vi "Modbus LDO Sensors.vi"(8 "error in":errorcluster, 11 "PLC Data":T1) -> (0 "error out":errorcluster, 3 "PLC Data Output":T1)   [LabVIEW 2020, in "Modbus.lvlib"]
uses:
  Modbus.lvlib
  Modbus PLC Data All.ctl
  Modbus FVIR Control.ctl
  Modbus LDO Control.ctl
  WritingDataFile/Data to Save.ctl
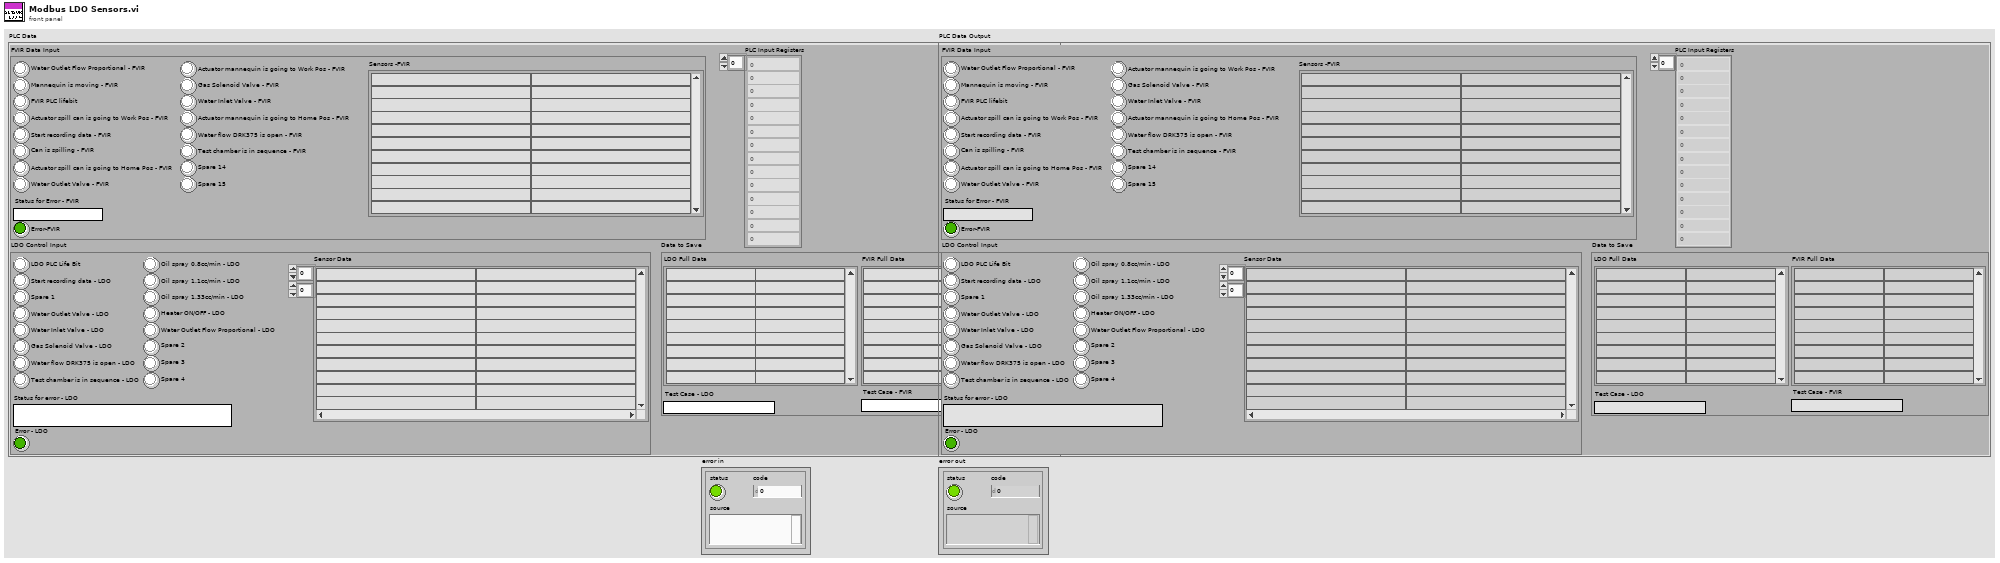
[diagram p1: front panel]
types:
  T1 = typedef "Modbus PLC Data All.ctl" = cluster{"FVIR Data Input":T2, "LDO Control Input":T3, "PLC Input Registers":u16[], "Data to Save":T4}
  T2 = typedef "Modbus FVIR Control.ctl" = cluster{"Spare 15":bool, "Spare 14":bool, "Actuator mannequin is going to Work Pos - FVIR":bool, "Actuator mannequin is going to Home Pos - FVIR":bool, "Test chamber is in sequence - FVIR ":bool, "Water flow DRK375 is open - FVIR":bool, "Gas Solenoid Valve - FVIR":bool, "Water Inlet Valve - FVIR":bool, "Water Outlet Flow Proportional - FVIR":bool, "Start recording data - FVIR":bool, "Actuator spill can is going to Work Pos - FVIR":bool, "Actuator spill can is going to Home Pos - FVIR":bool, "Water Outlet Valve - FVIR":bool, "Can is spilling - FVIR":bool, "Mannequin is moving - FVIR":bool, "FVIR PLC lifebit":bool, "Status for Error - FVIR":string, "Error-FVIR":bool, "Sensors -FVIR":string[][]}
  T3 = typedef "Modbus LDO Control.ctl" = cluster{"LDO PLC Life Bit":bool, "Start recording data - LDO":bool, "Spare 1":bool, "Water Outlet Valve - LDO":bool, "Water Inlet Valve - LDO":bool, "Gas Solenoid Valve - LDO":bool, "Water flow DRK375 is open - LDO":bool, "Test chamber is in sequence - LDO":bool, "Oil spray 0.8cc/min - LDO":bool, "Oil spray 1.1cc/min - LDO":bool, "Oil spray 1.33cc/min - LDO":bool, "Heater ON/OFF - LDO":bool, "Water Outlet Flow Proportional - LDO":bool, "Spare 2":bool, "Spare 3":bool, "Spare 4":bool, "Status for error - LDO":string, "Error - LDO":bool, "Sensor Data":string[][]}
  T4 = typedef "Data to Save.ctl" = cluster{"LDO Full Data":string[][], "FVIR Full Data":string[][], "Test Case - FVIR":string, "Test Case - LDO":string}
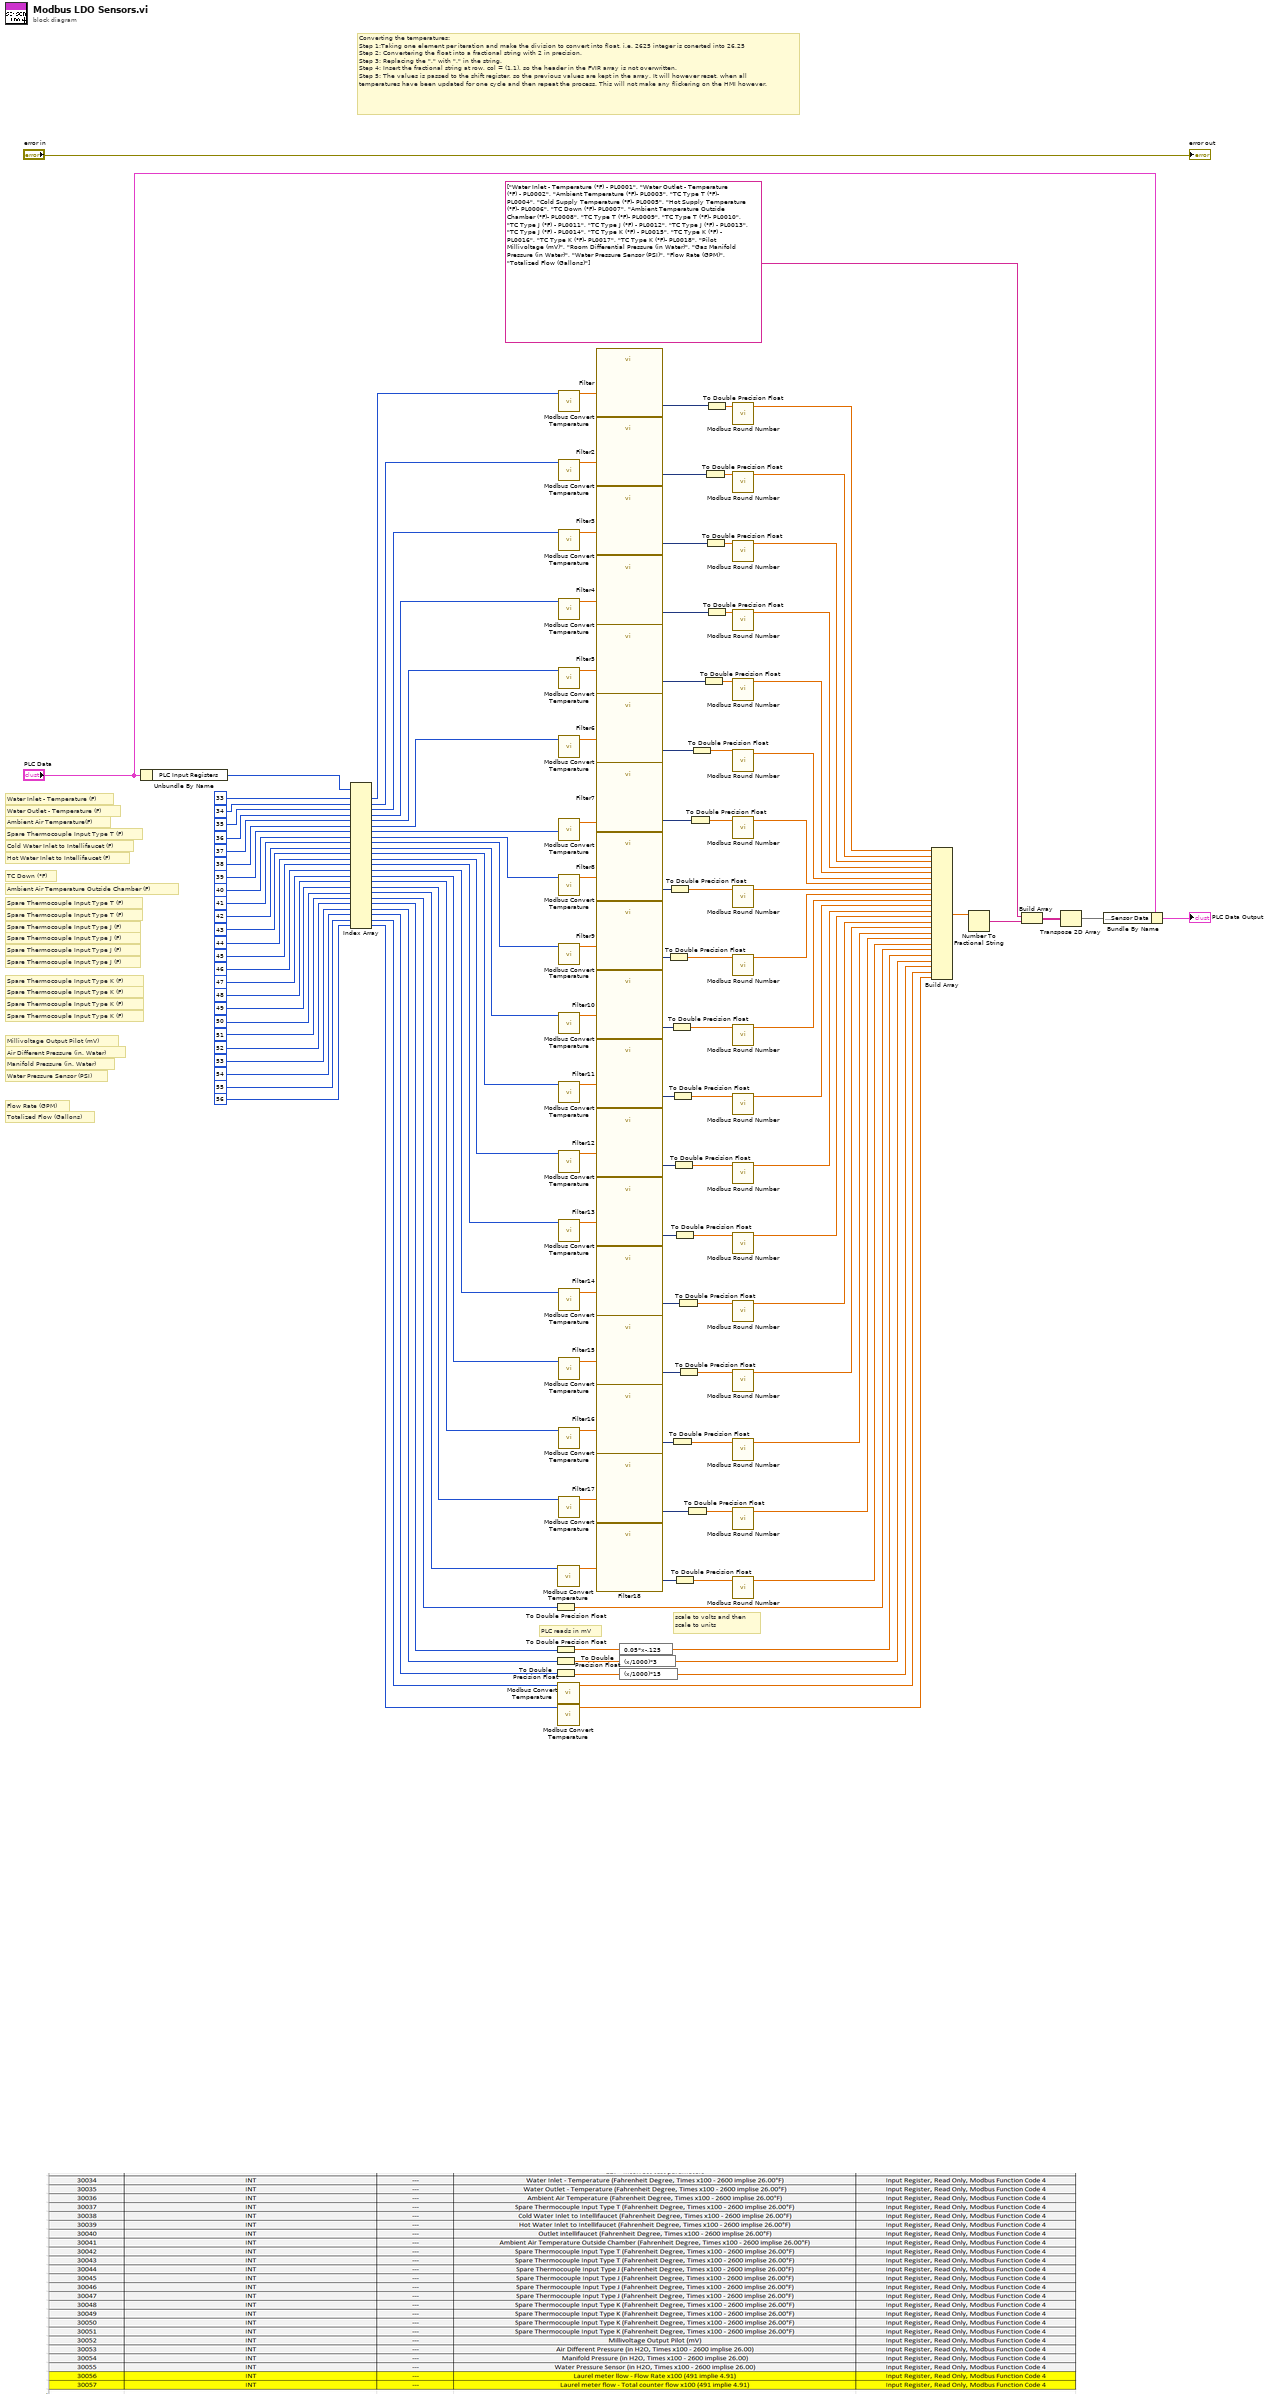
[diagram p0: block diagram]
diagram:
  # "scale to volts and then \nscale to units"
  # "PLC reads in mV"
  # "Totalized Flow (Gallons)"
  # "Flow Rate (GPM)"
  # "Water Pressure Sensor (PSI)"
  # "Manifold Pressure (in. Water)"
  # "Air Different Pressure (in. Water)"
  # "Millivoltage Output Pilot (mV)"
  # "Spare Thermocouple Input Type K (F)"
  # "Spare Thermocouple Input Type K (F)"
  # "Spare Thermocouple Input Type K (F)"
  # "Spare Thermocouple Input Type K (F)"
  # "Spare Thermocouple Input Type J (F)"
  # "Spare Thermocouple Input Type J (F)"
  # "Spare Thermocouple Input Type J (F)"
  # "Spare Thermocouple Input Type J (F)"
  # "Spare Thermocouple Input Type T (F)"
  # "Spare Thermocouple Input Type T (F)"
  # "Ambient Air Temperature Outside Chamber (F)"
  # "TC Down (°F)"
  # "Hot Water Inlet to Intellifaucet (F)"
  # "Cold Water Inlet to Intellifaucet (F)"
  # "Spare Thermocouple Input Type T (F)"
  # "Ambient Air Temperature(F)"
  # "Water Outlet - Temperature (F)"
  # "Water Inlet - Temperature (F)"
  # "Converting the temperatures: \nStep 1:Taking one element per iteration and make the division to convert into float, i.e. 2625 integer is conerted into 26,25\nStep 2: Convertering the float into a fractional string with 2 in precision. \nStep 3: Replacing the \",\" with \".\" in the string.\nStep 4: Insert the fractional string at row, col = (1,1), so the header in the FVIR array is not overwritten. \nStep 5: The values is passed to the shift register, so the previous values are kept in the array. It will however reset, when all temperatures have been updated for one cycle and then repeat the process. This will not make any flickering on the HMI however."
  n1 = Unbundle By Name("PLC Data") -> ("PLC Input Registers"=w82:u16[])
  n2 = Index Array(array=w82, index #1=33 ("index"), index #2=34 ("index"), index #3=35 ("index"), index #4=36 ("index"), index #5=37 ("index"), index #6=38 ("index"), index #7=39 ("index"), index #8=40 ("index"), index #9=41 ("index"), index #10=42 ("index"), index #11=43 ("index"), index #12=44 ("index"), index #13=45 ("index"), index #14=46 ("index"), index #15=47 ("index"), index #16=48 ("index"), index #17=49 ("index"), index #18=50 ("index"), index #19=51 ("index"), index #20=52 ("index"), index #21=53 ("index"), index #22=54 ("index"), index #23=55 ("index"), index #24=56 ("index")) -> (element #1=w114:u16, element #2=w113:u16, element #3=w112:u16, element #4=w111:u16, element #5=w110:u16, element #6=w109:u16, element #7=w108:u16, element #8=w107:u16, element #9=w106:u16, element #10=w105:u16, element #11=w104:u16, element #12=w103:u16, element #13=w102:u16, element #14=w101:u16, element #15=w100:u16, element #16=w99:u16, element #17=w98:u16, element #18=w97:u16, element #19=w74:u16, element #20=w95:u16, element #21=w81:u16, element #22=w94:u16, element #23=w93:u16, element #24=w92:u16)
  n3 = To Double Precision Float(number=w74) -> (double precision float=w73:dbl)
  n4 = To Double Precision Float(number=w95) -> (double precision float=w79:dbl)
  n5 = To Double Precision Float(number=w81) -> (double precision float=w80:dbl)
  n6 = To Double Precision Float(number=w94) -> (double precision float=w76:dbl)
  n7 = call "Modbus Convert Temperature.vi"("PLC Value"=w97) -> ("Converted Value"=w37:dbl)  [unwired: 9 in, 1 out]
  n8 = call "Modbus Convert Temperature.vi"("PLC Value"=w93) -> ("Converted Value"=w91:dbl)  [unwired: 9 in, 1 out]
  n9 = call "Modbus Convert Temperature.vi"("PLC Value"=w92) -> ("Converted Value"=w90:dbl)  [unwired: 9 in, 1 out]
  n10 = call "Modbus Convert Temperature.vi"("PLC Value"=w114) -> ("Converted Value"=w72:dbl)  [unwired: 9 in, 1 out]
  n11 = call "Modbus Convert Temperature.vi"("PLC Value"=w113) -> ("Converted Value"=w69:dbl)  [unwired: 9 in, 1 out]
  n12 = call "Modbus Convert Temperature.vi"("PLC Value"=w112) -> ("Converted Value"=w67:dbl)  [unwired: 9 in, 1 out]
  n13 = call "Modbus Convert Temperature.vi"("PLC Value"=w111) -> ("Converted Value"=w65:dbl)  [unwired: 9 in, 1 out]
  n14 = call "Modbus Convert Temperature.vi"("PLC Value"=w110) -> ("Converted Value"=w63:dbl)  [unwired: 9 in, 1 out]
  n15 = call "Modbus Convert Temperature.vi"("PLC Value"=w109) -> ("Converted Value"=w61:dbl)  [unwired: 9 in, 1 out]
  n16 = call "Modbus Convert Temperature.vi"("PLC Value"=w108) -> ("Converted Value"=w59:dbl)  [unwired: 9 in, 1 out]
  n17 = call "Modbus Convert Temperature.vi"("PLC Value"=w107) -> ("Converted Value"=w57:dbl)  [unwired: 9 in, 1 out]
  n18 = call "Modbus Convert Temperature.vi"("PLC Value"=w106) -> ("Converted Value"=w55:dbl)  [unwired: 9 in, 1 out]
  n19 = call "Modbus Convert Temperature.vi"("PLC Value"=w105) -> ("Converted Value"=w53:dbl)  [unwired: 9 in, 1 out]
  n20 = call "Modbus Convert Temperature.vi"("PLC Value"=w104) -> ("Converted Value"=w51:dbl)  [unwired: 9 in, 1 out]
  n21 = call "Modbus Convert Temperature.vi"("PLC Value"=w103) -> ("Converted Value"=w49:dbl)  [unwired: 9 in, 1 out]
  n22 = call "Modbus Convert Temperature.vi"("PLC Value"=w102) -> ("Converted Value"=w47:dbl)  [unwired: 9 in, 1 out]
  n23 = call "Modbus Convert Temperature.vi"("PLC Value"=w101) -> ("Converted Value"=w45:dbl)  [unwired: 9 in, 1 out]
  n24 = call "Modbus Convert Temperature.vi"("PLC Value"=w100) -> ("Converted Value"=w43:dbl)  [unwired: 9 in, 1 out]
  n25 = call "Modbus Convert Temperature.vi"("PLC Value"=w99) -> ("Converted Value"=w41:dbl)  [unwired: 9 in, 1 out]
  n26 = call "Modbus Convert Temperature.vi"("PLC Value"=w98) -> ("Converted Value"=w39:dbl)  [unwired: 9 in, 1 out]
  n27 = call "Filter"("Signal"=w72) -> ("Filtered Signal"=w71:dynamicdata)  [unwired: 9 in, 1 out]
  n28 = call "Filter2"("Signal"=w69) -> ("Filtered Signal"=w70:dynamicdata)  [unwired: 9 in, 1 out]
  n29 = call "Filter3"("Signal"=w67) -> ("Filtered Signal"=w68:dynamicdata)  [unwired: 9 in, 1 out]
  n30 = call "Filter4"("Signal"=w65) -> ("Filtered Signal"=w66:dynamicdata)  [unwired: 9 in, 1 out]
  n31 = call "Filter5"("Signal"=w63) -> ("Filtered Signal"=w64:dynamicdata)  [unwired: 9 in, 1 out]
  n32 = call "Filter6"("Signal"=w61) -> ("Filtered Signal"=w62:dynamicdata)  [unwired: 9 in, 1 out]
  n33 = call "Filter7"("Signal"=w59) -> ("Filtered Signal"=w60:dynamicdata)  [unwired: 9 in, 1 out]
  n34 = call "Filter8"("Signal"=w57) -> ("Filtered Signal"=w58:dynamicdata)  [unwired: 9 in, 1 out]
  n35 = call "Filter9"("Signal"=w55) -> ("Filtered Signal"=w56:dynamicdata)  [unwired: 9 in, 1 out]
  n36 = call "Filter10"("Signal"=w53) -> ("Filtered Signal"=w54:dynamicdata)  [unwired: 9 in, 1 out]
  n37 = call "Filter11"("Signal"=w51) -> ("Filtered Signal"=w52:dynamicdata)  [unwired: 9 in, 1 out]
  n38 = call "Filter12"("Signal"=w49) -> ("Filtered Signal"=w50:dynamicdata)  [unwired: 9 in, 1 out]
  n39 = call "Filter13"("Signal"=w47) -> ("Filtered Signal"=w48:dynamicdata)  [unwired: 9 in, 1 out]
  n40 = call "Filter14"("Signal"=w45) -> ("Filtered Signal"=w46:dynamicdata)  [unwired: 9 in, 1 out]
  n41 = call "Filter15"("Signal"=w43) -> ("Filtered Signal"=w44:dynamicdata)  [unwired: 9 in, 1 out]
  n42 = call "Filter16"("Signal"=w41) -> ("Filtered Signal"=w42:dynamicdata)  [unwired: 9 in, 1 out]
  n43 = call "Filter17"("Signal"=w39) -> ("Filtered Signal"=w40:dynamicdata)  [unwired: 9 in, 1 out]
  n44 = call "Filter18"("Signal"=w37) -> ("Filtered Signal"=w38:dynamicdata)  [unwired: 9 in, 1 out]
  n45 = expression code="0.05*x-.125"(w79) -> (w78:dbl)
  n46 = expression code="(x/1000)*3"(w80) -> (w77:dbl)
  n47 = expression code="(x/1000)*15"(w76) -> (w75:dbl)
  n48 = To Double Precision Float(number=w56) -> (double precision float=w20:dbl)
  n49 = To Double Precision Float(number=w58) -> (double precision float=w22:dbl)
  n50 = To Double Precision Float(number=w54) -> (double precision float=w18:dbl)
  n51 = To Double Precision Float(number=w42) -> (double precision float=w6:dbl)
  n52 = To Double Precision Float(number=w52) -> (double precision float=w16:dbl)
  n53 = To Double Precision Float(number=w50) -> (double precision float=w14:dbl)
  n54 = To Double Precision Float(number=w48) -> (double precision float=w12:dbl)
  n55 = To Double Precision Float(number=w38) -> (double precision float=w2:dbl)
  n56 = To Double Precision Float(number=w46) -> (double precision float=w10:dbl)
  n57 = To Double Precision Float(number=w44) -> (double precision float=w8:dbl)
  n58 = To Double Precision Float(number=w40) -> (double precision float=w4:dbl)
  n59 = To Double Precision Float(number=w60) -> (double precision float=w24:dbl)
  n60 = To Double Precision Float(number=w62) -> (double precision float=w26:dbl)
  n61 = To Double Precision Float(number=w64) -> (double precision float=w28:dbl)
  n62 = To Double Precision Float(number=w70) -> (double precision float=w34:dbl)
  n63 = To Double Precision Float(number=w68) -> (double precision float=w32:dbl)
  n64 = To Double Precision Float(number=w71) -> (double precision float=w36:dbl)
  n65 = To Double Precision Float(number=w66) -> (double precision float=w30:dbl)
  n66 = call "Modbus Round Number.vi"("Number"=w36) -> ("Rounded Number"=w35:dbl)  [unwired: 10 in]
  n67 = call "Modbus Round Number.vi"("Number"=w34) -> ("Rounded Number"=w33:dbl)  [unwired: 10 in]
  n68 = call "Modbus Round Number.vi"("Number"=w32) -> ("Rounded Number"=w31:dbl)  [unwired: 10 in]
  n69 = call "Modbus Round Number.vi"("Number"=w30) -> ("Rounded Number"=w29:dbl)  [unwired: 10 in]
  n70 = call "Modbus Round Number.vi"("Number"=w28) -> ("Rounded Number"=w27:dbl)  [unwired: 10 in]
  n71 = call "Modbus Round Number.vi"("Number"=w26) -> ("Rounded Number"=w25:dbl)  [unwired: 10 in]
  n72 = call "Modbus Round Number.vi"("Number"=w24) -> ("Rounded Number"=w23:dbl)  [unwired: 10 in]
  n73 = call "Modbus Round Number.vi"("Number"=w22) -> ("Rounded Number"=w21:dbl)  [unwired: 10 in]
  n74 = call "Modbus Round Number.vi"("Number"=w20) -> ("Rounded Number"=w19:dbl)  [unwired: 10 in]
  n75 = call "Modbus Round Number.vi"("Number"=w18) -> ("Rounded Number"=w17:dbl)  [unwired: 10 in]
  n76 = call "Modbus Round Number.vi"("Number"=w16) -> ("Rounded Number"=w15:dbl)  [unwired: 10 in]
  n77 = call "Modbus Round Number.vi"("Number"=w14) -> ("Rounded Number"=w13:dbl)  [unwired: 10 in]
  n78 = call "Modbus Round Number.vi"("Number"=w12) -> ("Rounded Number"=w11:dbl)  [unwired: 10 in]
  n79 = call "Modbus Round Number.vi"("Number"=w10) -> ("Rounded Number"=w9:dbl)  [unwired: 10 in]
  n80 = call "Modbus Round Number.vi"("Number"=w8) -> ("Rounded Number"=w7:dbl)  [unwired: 10 in]
  n81 = call "Modbus Round Number.vi"("Number"=w6) -> ("Rounded Number"=w5:dbl)  [unwired: 10 in]
  n82 = call "Modbus Round Number.vi"("Number"=w4) -> ("Rounded Number"=w3:dbl)  [unwired: 10 in]
  n83 = call "Modbus Round Number.vi"("Number"=w2) -> ("Rounded Number"=w1:dbl)  [unwired: 10 in]
  n84 = Build Array(w35, w33, w31, w29, w27, w25, w23, w21, w19, w17, w15, w13, w11, w9, w7, w5, w3, w1, w73, w78, w77, w75, w91, w90) -> (w89:dbl[])
  n85 = Number To Fractional String(number=w89) -> (F-format string=w88:string[])  [unwired: 3 in]
  n86 = Build Array(string[] ["Water Inlet - Temperature (°F) - PL0001", "Water Outlet - Temperature (°F) - PL0002", "Ambient Temperature (°F)- PL0003", "TC Type T (°F)- PL0004", "Cold Supply Temperature (°F)- PL0005", "Hot Supply Temperature (°F)- PL0006", "TC Down (°F)- PL0007", "Ambient Temperature Outside Chamber (°F)- PL0008", "TC Type T (°F)- PL0009", "TC Type T (°F)- PL0010", "TC Type J (°F) - PL0011", "TC Type J (°F) - PL0012", "TC Type J (°F) - PL0013", "TC Type J (°F) - PL0014", "TC Type K (°F) - PL0015", "TC Type K (°F) - PL0016", "TC Type K (°F)- PL0017", "TC Type K (°F)- PL0018", "Pilot Millivoltage (mV)", "Room Differential Pressure (in Water)", "Gas Manifold Pressure (in Water)", "Water Pressure Sensor (PSI)", "Flow Rate (GPM)", "Totalized Flow (Gallons)"] ("Array 2"), w88) -> (w86:string[][])
  n87 = Transpose 2D Array(2D array=w86) -> (transposed array=w85:string[][])
  n88 = Bundle By Name(cluster="PLC Data", "LDO Control Input.Sensor Data"=w85) -> (→"PLC Data Output":T1)
  "error out" <- "error in"
